vi "Actor Core.vi"(8 "error in":errorcluster, 11 "Measure Object in":refnum<class "Spectrum Recorder.lvclass">) -> (0 "error out":errorcluster, 3 "Actor out":refnum<class "Actor.lvclass">)   [LabVIEW 2016]
doc: "(<B>Filename</B>: Actor Framework.lvlib:Actor.lvclass:Actor Core.vi)\n\nReceives messages to the actor, reacts to them, and initiates any error handling that may shut the actor down.\n\nDescendant classes may override this VI to append parallel tasks for the actor to complete while it handles messages. Overrides use the Call Parent Method node."
uses:
  Spectrum Recorder.lvclass
  <vilib>/ActorFramework/Actor/Actor.lvclass
  <vilib>/ActorFramework/Stop Msg/Stop Msg.lvclass
  Measure_core/Worker Messages/Initialize Work Msg/Initialize Work Msg.lvclass
  Measure_core/Template Module Messages/Result Reply Msg/Result Reply Msg.lvclass
  Measure_core/Worker Messages/Stop Work Msg/Stop Work Msg.lvclass
  C:/github/Measure_core/Sequence Elements/Sweep Sequence/Sweep.lvclass
  C:/github/Measure_core/Sequence Elements/Sequence Element/Sequence Element.lvclass
  C:/github/Measure_core/Worker/Worker.lvclass
  C:/github/Measure_core/Template Module/Template Module.lvclass
  C:/Program Files/National Instruments/LabVIEW 2016/vi.lib/ActorFramework/Actor/Actor.lvclass
  Spectrum Recorder Configuration.ctl
panel:
  out "Spectrum plot":cluster{dbl[], dbl[]}[](graph)
  out "Data file path":path=path "C:/Data"
  out "State":bool
  in  "Exit":bool
  in  "Stop":bool
  in  "Open digitizer":bool
  in  "Configuration":T1={"Start"=500000.0, "End"=2000000.0, "Duration"=40.0, "Filter time constant"=0.004, "Repeat (-1: forever)"=1, "Update rate"=1.0, "Data storage folder"=path "C:/Data"} {"Update rate" min=0.001 max=10.0 step=0.001 format="%#_6ps"; "Repeat (-1: forever)" format="%.0p"; "Filter time constant" format="%#_6ps"; "Duration" format="%#_6ps"; "End" format="%#_6pHz"; "Start" format="%#_6pHz"}
  in  "Record":bool
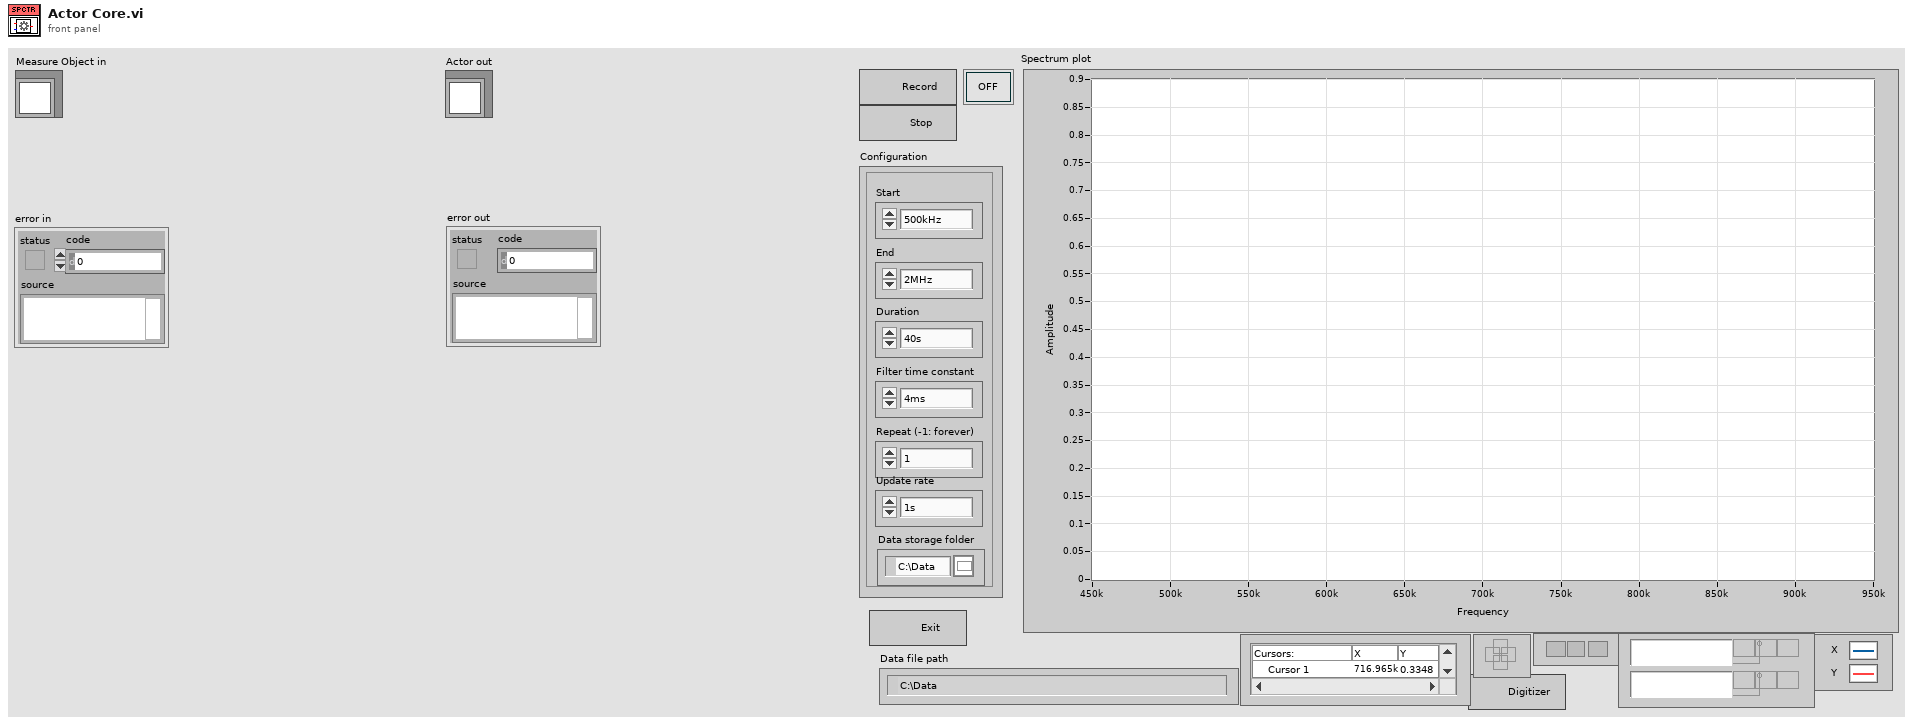
[diagram p1: front panel]
types:
  T1 = typedef "Spectrum Recorder Configuration.ctl" = cluster{"Start":dbl, "End":dbl, "Duration":dbl, "Filter time constant":dbl, "Repeat (-1: forever)":i32, "Update rate":dbl, "Data storage folder":path}
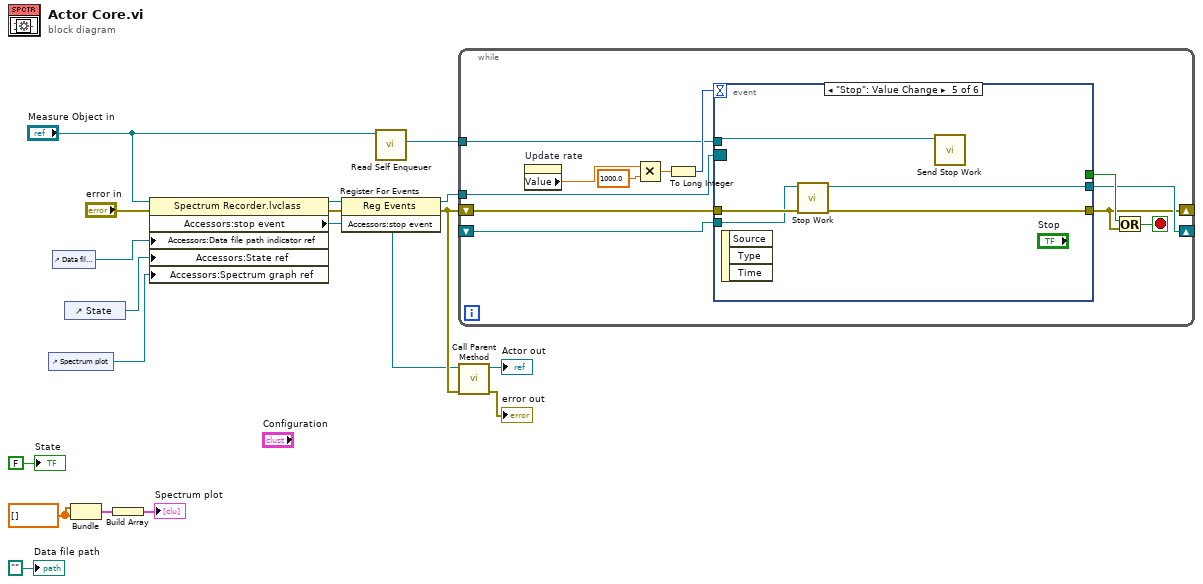
[diagram p0: block diagram]
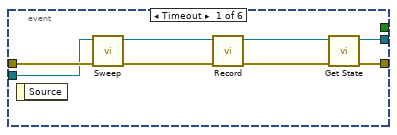
[diagram p2: hidden frame]
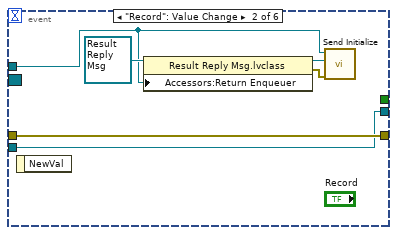
[diagram p3: hidden frame]
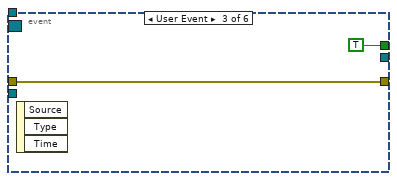
[diagram p4: hidden frame]
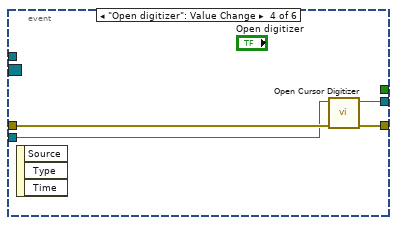
[diagram p5: hidden frame]
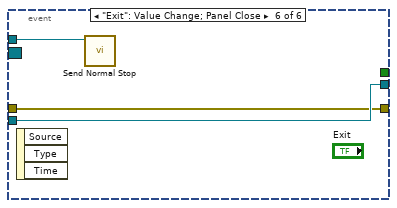
[diagram p6: hidden frame]
diagram:
  w9 = dbl[] []
  n1 = control-ref of="Spectrum plot"() -> (w6:refnum<vi>)
  n2 = control-ref of="Data file path"() -> (w8:refnum<vi>)
  n3 = control-ref of="State"() -> (w7:refnum<vi>)
  n4 = Bundle(w9, w9) -> (w10:cluster{dbl[], dbl[]})  [unwired: 1 in]
  n5 = Build Array(w10) -> (→"Spectrum plot":cluster{dbl[], dbl[]}[])
  n6 = property class="Spectrum Recorder.lvclass"(reference="Measure Object in", error in="error in", "Accessors:Data file path indicator ref"=w8, "Accessors:State ref"=w7, "Accessors:Spectrum graph ref"=w6) -> (reference out=w2:refnum<class "Spectrum Recorder.lvclass">, error out=w3:errorcluster, "Accessors:stop event"=w4:refnum<user-event>)
  n7 = register-events(error in=w3, w4) -> (reference out=w15:refnum<event-registration>, error out=w16:errorcluster)  [unwired: 1 in]
  n8 = call <vilib>:"Read Self Enqueuer.vi"("Actor"="Measure Object in") -> ("Self Enqueuer"=w14:refnum<class "Message Enqueuer.lvclass">)  [unwired: 10 in]
  n9 = while {
    shift-right: [w24] -> _
    shift-left: _ -> [w25]
    shift-right: [w21] -> _
    shift-left: w16 -> [w23]
    tunnel: w15 -> [w20]
    tunnel: w14 -> [w19]
    stop <- w22 stop-if-true
    n10 = property on="Update rate" class="DigNum (strict)"() -> ("Value"=w29:dbl)  [unwired: 2 in, 2 out]
    n11 = Multiply(x=w29, y=1000.0) -> (x*y=w27:dbl)
    n12 = To Long Integer(number=w27) -> (32bit integer=w26:i32)
    n13 = event shown="[4] \"Stop\": Value Change" {
      selector: w20 -> [_ _ _ _ _ _]
      dyn-events: _ -> [_ _ _ _ _ _]
      timeout: w26 -> [_ _ _ _ _ _]
      tunnel: [_ _ TRUE ("Exit") _ _ _] -> w30
      tunnel: w25 -> [w36 w43 _ w48 w54 w58]
      tunnel: [w31 w43 _ w47 w52 w58] -> w24
      tunnel: w23 -> [w38 w44 w45 w50 w55 w57]
      tunnel: [w33 w44 w45 w49 w53 w57] -> w21
      tunnel: w19 -> [_ w40 _ _ w51 w56]
      event Timeout {
        n14 = event-data() -> ()  [unwired: 1 in, 1 out]
        n15 = call-dynamic "Sweep.vi"("error in (no error)"=w38, "Spectrum Recorder in"=w36) -> ("error out"=w37:errorcluster, "Spectrum Recorder out"=w34:refnum<class "Spectrum Recorder.lvclass">)  [unwired: 8 in]
        n16 = call-dynamic "Record.vi"("error in (no error)"=w37, "Spectrum Recorder in"=w34) -> ("error out"=w35:errorcluster, "Spectrum Recorder out"=w32:refnum<class "Spectrum Recorder.lvclass">)  [unwired: 8 in]
        n17 = call-dynamic "Get State.vi"("error in (no error)"=w35, "Spectrum Recorder in"=w32) -> ("error out"=w33:errorcluster, "Spectrum Recorder out"=w31:refnum<class "Spectrum Recorder.lvclass">)  [unwired: 8 in]
      }
      event "Record": Value Change {
        n18 = event-data() -> ()  [unwired: 1 in, 1 out]
        n19 = property class="Result Reply Msg.lvclass"(reference=refnum<class "Result Reply Msg.lvclass"> refnum ("Reply to"), "Accessors:Return Enqueuer"=w40) -> (reference out=w41:refnum<class "Result Reply Msg.lvclass">, error out=w39:errorcluster)  [unwired: 1 in]
        n20 = call "Send Initialize.vi"("error in (no error)"=w39, "Reply to"=w41, "Message Enqueuer"=w40) -> ()  [unwired: 7 in, 2 out]
      }
      event User Event {
        n21 = event-data() -> ()  [unwired: 1 in, 3 out]
      }
      event "Open digitizer": Value Change {
        n22 = event-data() -> ()  [unwired: 1 in, 3 out]
        n23 = call-dynamic "Open Cursor Digitizer.vi"("error in (no error)"=w50, "Spectrum Recorder in"=w48) -> ("error out"=w49:errorcluster, "Spectrum Recorder out"=w47:refnum<class "Spectrum Recorder.lvclass">)  [unwired: 8 in]
      }
      event "Stop": Value Change {
        n24 = event-data() -> ()  [unwired: 1 in, 3 out]
        n25 = call-dynamic "Stop Work.vi"("error in (no error)"=w55, "Spectrum Recorder in"=w54) -> ("error out"=w53:errorcluster, "Spectrum Recorder out"=w52:refnum<class "Spectrum Recorder.lvclass">)  [unwired: 8 in]
        n26 = call "Send Stop Work.vi"("Message Enqueuer"=w51) -> ()  [unwired: 9 in, 2 out]
      }
      event "Exit": Value Change; Panel Close {
        n27 = event-data() -> ()  [unwired: 1 in, 3 out]
        n28 = call <vilib>:"Send Normal Stop.vi"("Message Enqueuer"=w56) -> ()  [unwired: 10 in, 1 out]
      }
    }
    n29 = Or(x=w30, y=w21) -> (x .or. y?=w22:bool)
  }
  n30 = call-parent "Call Parent Method"("error in"=w16, "Measure Object in"=w2) -> ("error out"=→"error out":errorcluster, "Actor out"=→"Actor out":refnum<class "Actor.lvclass">)  [unwired: 8 in]
  "Data file path" <- path ""
  "State" <- FALSE ("State")
